vi "cvt.vi"(7 "LWSR":refnum<class "Web Request.lvclass">, 11 "force":u8) -> ()   [LabVIEW 2014]
uses:
  <vilib>/wsapi/Web Request.lvclass
  Controller/Controller.lvclass
panel:
  out "String":string
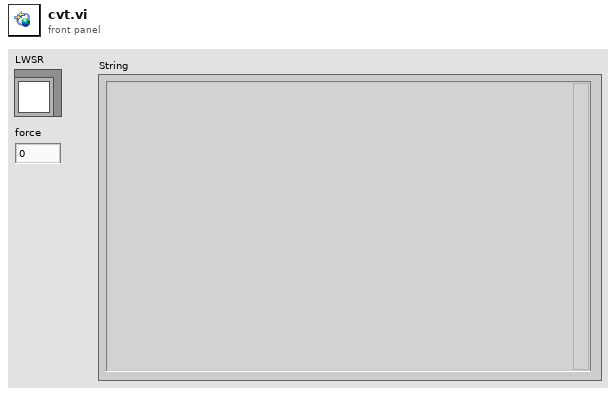
[diagram p1: front panel]
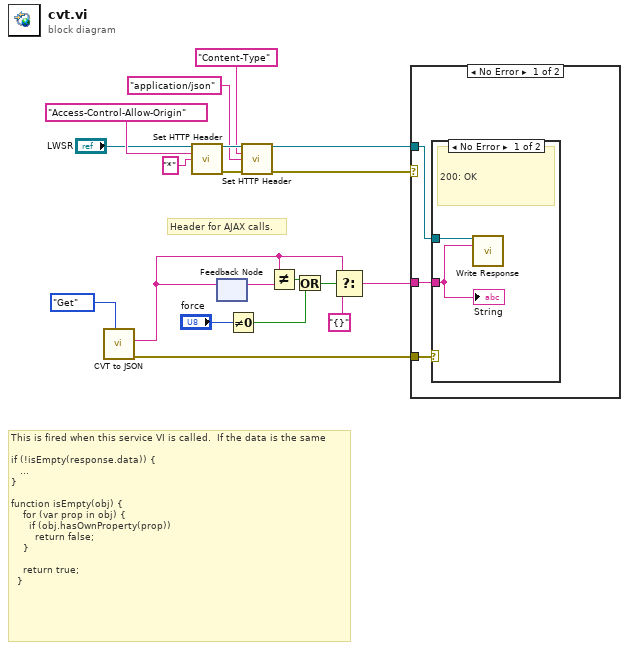
[diagram p0: block diagram]
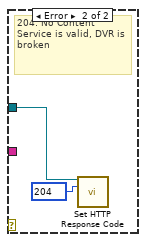
[diagram p2: hidden frame]
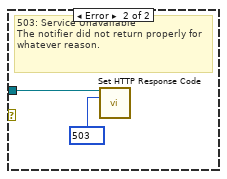
[diagram p3: hidden frame]
diagram:
  # "This is fired when this service VI is called.  If the data is the same \n\nif (!isEmpty(response.data)) {\n   ...\n}\n\nfunction isEmpty(obj) {\n    for (var prop in obj) {\n      if (obj.hasOwnProperty(prop))\n        return false;\n    }\n\n    return true;\n  }"
  # "Header for AJAX calls."
  n1 = call "CVT to JSON.vi"("Select"=enum16{"Init", "Get", "Destroy"}."Get") -> ("error out"=w10:errorcluster, "json cvt"=w5:string)  [unwired: 8 in, 1 out]
  n2 = call <vilib>:"Set HTTP Header.vi"("LabVIEW Web Service Request"="LWSR", "header"="Access-Control-Allow-Origin", "header value"="*") -> ("LabVIEW Web Service Request out"=w17:refnum<class "Web Request.lvclass">, "error out"=w16:errorcluster)  [unwired: 11 in]
  n3 = feedback-in #1(w5) -> ()
  n4 = feedback #1() -> (w7:string)  [unwired: 1 in]
  n5 = Not Equal To 0?(x="force") -> (x != 0?=w1:bool)
  n6 = call <vilib>:"Set HTTP Header.vi"("LabVIEW Web Service Request"=w17, "header"="Content-Type", "header value"="application/json", "error in (no error)"=w16) -> ("LabVIEW Web Service Request out"=w12:refnum<class "Web Request.lvclass">, "error out"=w11:errorcluster)  [unwired: 10 in]
  n7 = Not Equal?(x=w5, y=w7) -> (x != y?=w8:bool)
  n8 = Or(x=w8, y=w1) -> (x .or. y?=w6:bool)
  n9 = Select(t=w5, s=w6, f="{}") -> (s? t:f=w3:string)
  n10 = case shown="No Error" w11 {
    tunnel: w10 -> [w22 _]
    tunnel: w12 -> [w21 w28]
    tunnel: w3 -> [w20 _]
    frame No Error {
      n11 = case shown="No Error" w22 {
        tunnel: w21 -> [w24 w26]
        tunnel: w20 -> [w23 _]
        frame No Error {
          # "200: OK"
          n12 = call <vilib>:"Write Response.vi"("LabVIEW Web Service Request"=w24, "response string"=w23) -> ()  [unwired: 12 in, 2 out]
          "String" <- w23
        }
        frame Error {
          w25 = 204 items=["100"=100, "101"=101, "200"=200, "201"=201, "202"=202, "203"=203, "204"=204, "205"=205, "206"=206, "300"=300, "301"=301, "302"=302, "303"=303, "304"=304, "305"=305, "306"=306, "307"=307, "400"=400, "401"=401, "402"=402, "403"=403, "404"=404, "405"=405, "406"=406, "407"=407, "408"=408, "409"=409, "410"=410, "411"=411, "412"=412, "413"=413, "414"=414, "415"=415, "416"=416, "417"=417, "500"=500, "501"=501, "502"=502, "503"=503, "504"=504, "505"=505] ("response code (200)")
          # "204: No Content\nService is valid, DVR is broken"
          n13 = call <vilib>:"Set HTTP Response Code.vi"("LabVIEW Web Service Request"=w26, "response code (200)"=w25) -> ()  [unwired: 12 in, 2 out]
        }
      }
    }
    frame Error {
      w27 = 503 items=["100"=100, "101"=101, "200"=200, "201"=201, "202"=202, "203"=203, "204"=204, "205"=205, "206"=206, "300"=300, "301"=301, "302"=302, "303"=303, "304"=304, "305"=305, "306"=306, "307"=307, "400"=400, "401"=401, "402"=402, "403"=403, "404"=404, "405"=405, "406"=406, "407"=407, "408"=408, "409"=409, "410"=410, "411"=411, "412"=412, "413"=413, "414"=414, "415"=415, "416"=416, "417"=417, "500"=500, "501"=501, "502"=502, "503"=503, "504"=504, "505"=505] ("response code (200)")
      # "503: Service Unavailable\nThe notifier did not return properly for whatever reason."
      n14 = call <vilib>:"Set HTTP Response Code.vi"("LabVIEW Web Service Request"=w28, "response code (200)"=w27) -> ()  [unwired: 12 in, 2 out]
    }
  }
